vi "subTiE_SetZEscape.vi"(5 "Wait for a second? (F)":bool, 6 "Ref":T2 caption="Ref (can be hidden)", 7 "TI-Ctrl":T1={"Obj"=5, "Cube Bottom"=5, "Cube Top"=1, "PFS-Ctrl"={"PFS IO"=FALSE, "PSF Err"=FALSE, "PSF Pos"=0}, "Z-Ctrl"={"Z-pos"=499.875, "Home"=FALSE, "Sensitivity"=1}, "Condenser"=2, "Lightpath"=enum."EYE"} {"Condenser" items=["A"=1, "DICN2"=2, "- empty 3 -"=3, "- empty 4 -"=4, "- empty 5 -"=5, "- empty 6 -"=6]; "Z-Ctrl"."Sensitivity" min=1 max=3 step=1 scale=1.0..3.0; "PFS-Ctrl"."PSF Pos" scale=0.0..16400.0; "Cube Top" items=["Quad-O"=1, "Quad-R"=2, "empty"=3, "empty"=4, "empty"=5, "DIC"=6]; "Cube Bottom" items=["Cy5"=1, "RFP"=2, "mO2"=3, "empty"=4, "CFP"=5, "GFP"=6]; "Obj" items=["20x/.75 Dry PFS"=1, "40x/1.3 Oil PFS"=2, "60x/1.4 Oil PFS"=3, "- empty 4 -"=4, "- empty 5 -"=5, "- empty 6 -"=6]}, 8 "error in":errorcluster) -> (0 "error out":errorcluster)   [LabVIEW 2015]
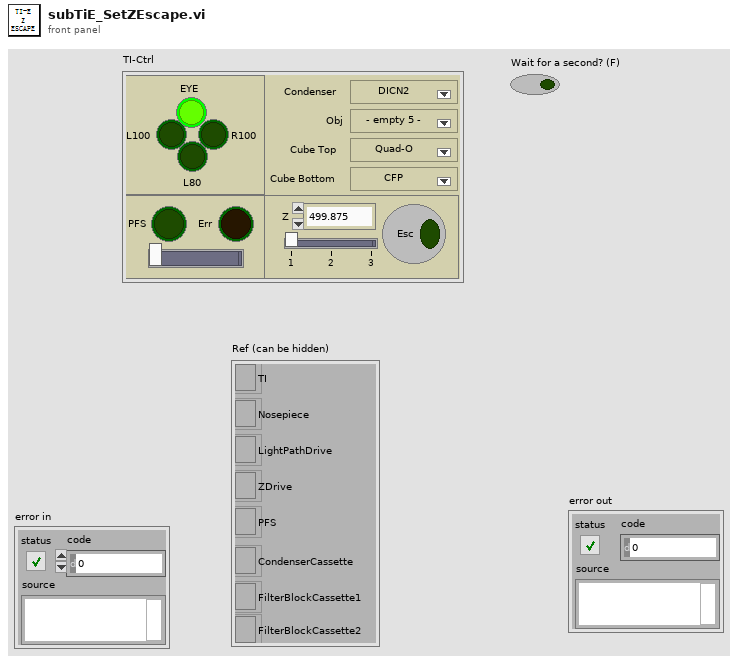
[diagram p1: front panel]
types:
  T1 = cluster{"Obj":u16, "Cube Bottom":u16, "Cube Top":u16, "PFS-Ctrl":cluster{"PFS IO":bool, "PSF Err":bool, "PSF Pos":u32}, "Z-Ctrl":cluster{"Z-pos":dbl, "Home":bool, "Sensitivity":u8}, "Condenser":u16, "Lightpath":enum32{"EYE", "L100", "R100", "L80"}}
  T2 = cluster{"TI":refnum<k7>, "Nosepiece":refnum<k7>, "LightPathDrive":refnum<k7>, "ZDrive":refnum<k7>, "PFS":refnum<k7>, "CondenserCassette":refnum<k7>, "FilterBlockCassette1":refnum<k7>, "FilterBlockCassette2":refnum<k7>}
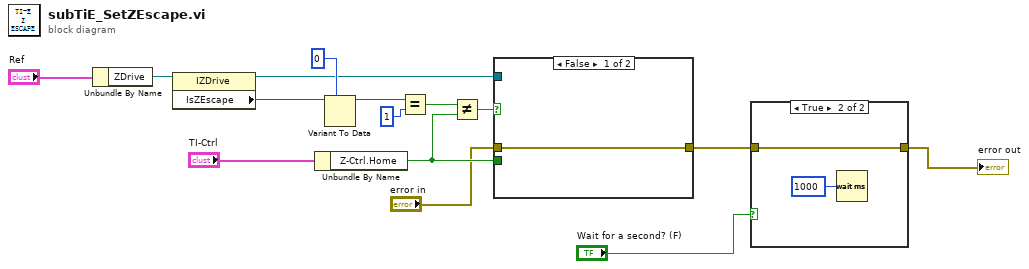
[diagram p0: block diagram]
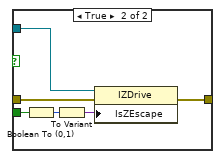
[diagram p3: hidden frame]
diagram:
  n1 = Unbundle By Name("Ref") -> ("ZDrive"=w15:refnum<k7>)
  n2 = property class="IZDrive"(reference=w15) -> (reference out=w7:refnum<k7>, "IsZEscape"=w10:variant)  [unwired: 1 in, 1 out]
  n3 = Unbundle By Name("TI-Ctrl") -> ("Z-Ctrl.Home"=w14:bool)
  n4 = Variant To Data(type=0, Variant=w10) -> (data=w12:i32)  [unwired: 1 in, 1 out]
  n5 = Equal?(x=w12, y=1) -> (x = y?=w9:bool)
  n6 = Not Equal?(x=w9, y=w14) -> (x != y?=w8:bool)
  n7 = case shown="False" w8 {
    tunnel: w14 -> [_ w20]
    tunnel: w7 -> [_ w19]
    tunnel: "error in" -> [w16 w18]
    tunnel: [w16 w17] -> w2
    frame False {
    }
    frame True {
      n8 = Boolean To (0,1)(Boolean=w20) -> (0, 1=w22:i16)
      n9 = To Variant(anything=w22) -> (Variant=w21:variant)
      n10 = property class="IZDrive"(reference=w19, error in=w18, "IsZEscape"=w21) -> (error out=w17:errorcluster)  [unwired: 1 out]
    }
  }
  n11 = case shown="True" "Wait for a second? (F)" {
    tunnel: w2 -> [w23 w25]
    tunnel: [w23 w25] -> w1
    frame False {
    }
    frame True {
      n12 = Wait (ms)(milliseconds to wait=u32 1000) -> ()  [unwired: 1 out]
    }
  }
  "error out" <- w1
